vi "Read from TDMS.vi"(8 "error in (no error)":errorcluster, 11 "Scan Data Process in":T1) -> (0 "error out":errorcluster, 3 "Scan Data Process out":T1)   [LabVIEW 2015, in "Exposure Process.lvlib"]
uses:
  Exposure Process.lvlib
  Control_Scan Data Process.ctl
  <vilib>/addons/PointValueMap/controls/PointMap.ctl
  Control_EXP Information.ctl
  Control_File Save Setup.ctl
  Control_Enable and Path.ctl
  Control_ICM Export Setting.ctl
  <vilib>/addons/PointValueMap/PointValueMap.lvlib
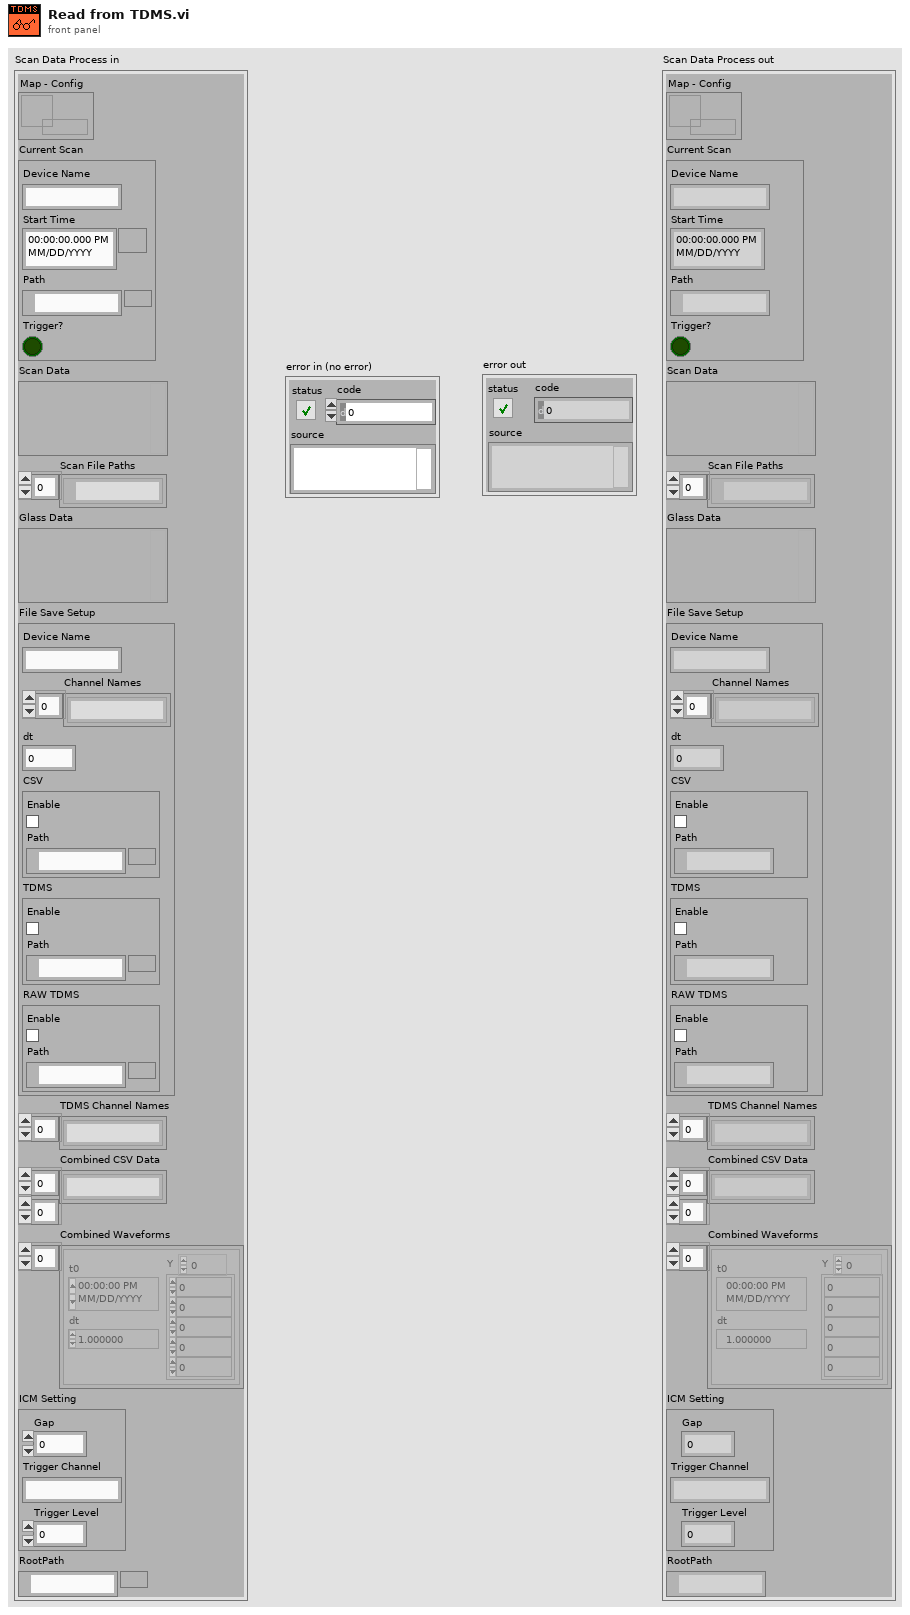
[diagram p1: front panel]
types:
  T1 = typedef "Exposure Process.lvlib/Control_Scan Data Process.ctl" = cluster{"Map - Config":T2, "Current Scan":T3, "Scan Data":variant, "Scan File Paths":path[], "Glass Data":variant, "File Save Setup":T4, "TDMS Channel Names":string[], "Combined CSV Data":string[][], "Combined Waveforms":waveform(dbl)[], "ICM Setting":T6, "RootPath":path}
  T2 = typedef "PointValueMap.lvlib/PointMap.ctl" = refnum<data-value>
  T3 = typedef "Exposure Process.lvlib/Control_EXP Information.ctl" = cluster{"Device Name":string, "Start Time":timestamp, "Path":path, "Trigger?":bool}
  T4 = typedef "Exposure Process.lvlib/Control_File Save Setup.ctl" = cluster{"Device Name":string, "Channel Names":string[], "dt":dbl, "CSV":T5, "TDMS":T5, "RAW TDMS":T5}
  T5 = typedef "Exposure Process.lvlib/Control_Enable and Path.ctl" = cluster{"Enable":bool, "Path":path}
  T6 = typedef "Exposure Process.lvlib/Control_ICM Export Setting.ctl" = cluster{"Gap":dbl, "Trigger Channel":string, "Trigger Level":dbl}
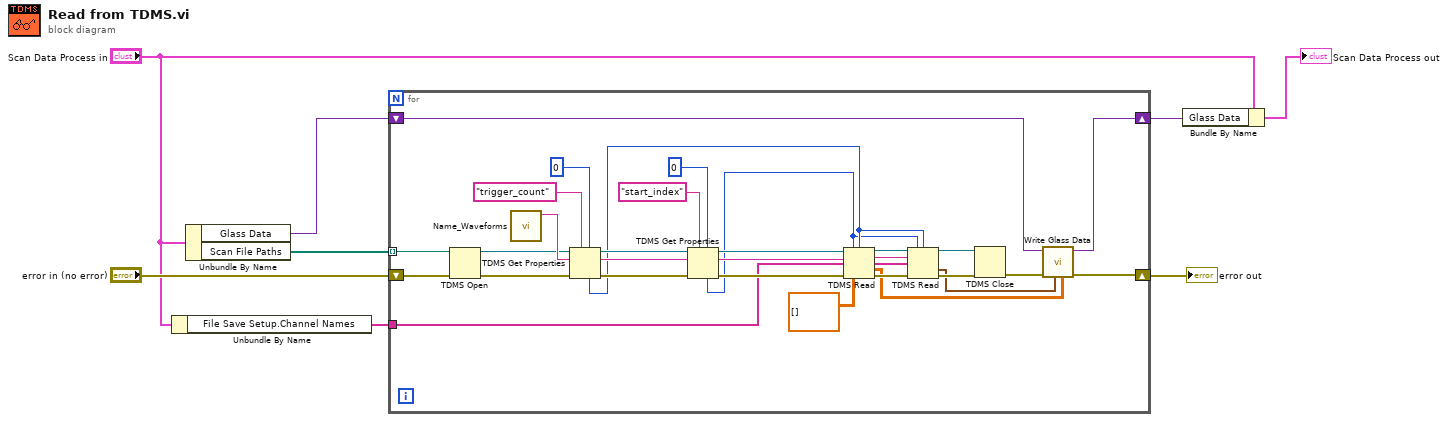
[diagram p0: block diagram]
diagram:
  n1 = Unbundle By Name("Scan Data Process in") -> ("File Save Setup.Channel Names"=w5:string[])
  n2 = Unbundle By Name("Scan Data Process in") -> ("Glass Data"=w4:variant, "Scan File Paths"=w6:path[])
  n3 = for {
    shift-right: [w14] -> w7
    shift-left: "error in (no error)" -> [w20]
    tunnel: w6 -> [w19] mode=indexing
    shift-right: [w12] -> w3
    shift-left: w4 -> [w13]
    tunnel: w5 -> [w18]
    n4 = TDMS Open(8:w20, 11:w19) -> (0:w21:errorcluster, 3:w9:refnum<k34>)  [unwired: 5 in]
    n5 = call "Name_Waveforms.vi"() -> ("Name"=w34:string)  [unwired: 11 in]
    n6 = TDMS Get Properties(5:i64 0, 7:"trigger_count", 8:w21, 10:w34, 11:w9) -> (0:w32:errorcluster, 2:w33:string, 3:w35:refnum<k34>, 4:w28:i64)  [unwired: 1 in, 2 out]
    n7 = TDMS Get Properties(5:i64 0, 7:"start_index", 8:w32, 10:w33, 11:w35) -> (0:w29:errorcluster, 2:w30:string, 3:w31:refnum<k34>, 4:w27:i64)  [unwired: 1 in, 2 out]
    n8 = TDMS Read(0:w31, 1:w27, 2:w28, 5:w30, 7:w18, 11:w29, 12:dbl[][] []) -> (4:w26:refnum<k34>, 6:w24:string, 8:w23:string[], 10:w10:dbl[][], 15:w25:errorcluster)  [unwired: 1 in, 1 out]
    n9 = TDMS Read(0:w26, 1:w27, 2:w28, 5:w24, 7:w23, 11:w25) -> (4:w17:refnum<k34>, 10:w11:waveform(dbl)[], 15:w16:errorcluster)  [unwired: 2 in, 3 out]
    n10 = TDMS Close(8:w16, 11:w17) -> (0:w15:errorcluster)  [unwired: 1 out]
    n11 = call "Write Glass Data.vi"("DBL Array"=w10, "Waveforms"=w11, "error in"=w15, "Glass Data in"=w13) -> ("error out"=w14:errorcluster, "Glass Data out"=w12:variant)  [unwired: 6 in]
  }
  "error out" <- w7
  n12 = Bundle By Name(cluster="Scan Data Process in", "Glass Data"=w3) -> (→"Scan Data Process out":T1)
